vi "Open PDF.vi"(4 "error in (no error)":errorcluster, 7 "Path":path) -> (0 "error out":errorcluster, 2 "Cancelled":bool)   [LabVIEW 2015]
doc: "This VI opens a Acrobat Reader (.pdf) document in an external instance of Acrobat Reader.\nWire the path to the Acrobat Reader document to the Path input.\nIf this is left unwired this VI will prompt for the document."
uses:
  <vilib>/registry/registry.llb/Registry RtKey.ctl
  <vilib>/registry/registry.llb/Registry SAM.ctl
  <vilib>/registry/registry.llb/Read Registry Value Simple STR.vi
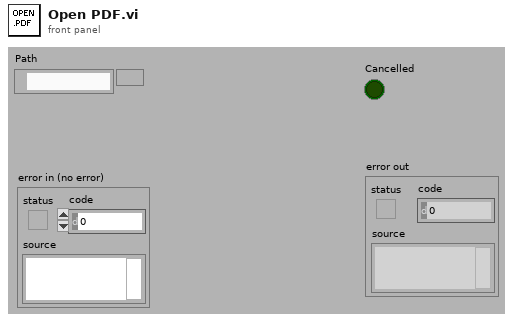
[diagram p1: front panel]
types:
  T1 = enum32{"existing file", "new file", "new or existing file", "existing dir", "new dir", "new or existing dir", "existing file (use LLBs)", "new file (use LLBs)", "new or existing file (use LLBs)", "new or existing file or directory (use LLBs)"}
  T2 = typedef "Registry SAM.ctl" = enum32{"KEY_QUERY_VALUE", "KEY_SET_VALUE", "KEY_CREATE_SUB_KEY", "KEY_ENUMERATE_SUB_KEYS", "KEY_NOTIFY", "KEY_CREATE_LINK", "KEY_READ", "KEY_WRITE", "KEY_ALL_ACCESS", "KEY_READ | KEY_WRITE"}
  T3 = typedef "Registry RtKey.ctl" = enum32{"HKEY_CLASSES_ROOT", "HKEY_CURRENT_USER", "HKEY_LOCAL_MACHINE", "HKEY_USERS", "HKEY_PERFORMANCE_DATA", "HKEY_CURRENT_CONFIG", "HKEY_DYN_DATA"}
  T4 = typedef "Registry refnum.ctl" = refnum<k1>
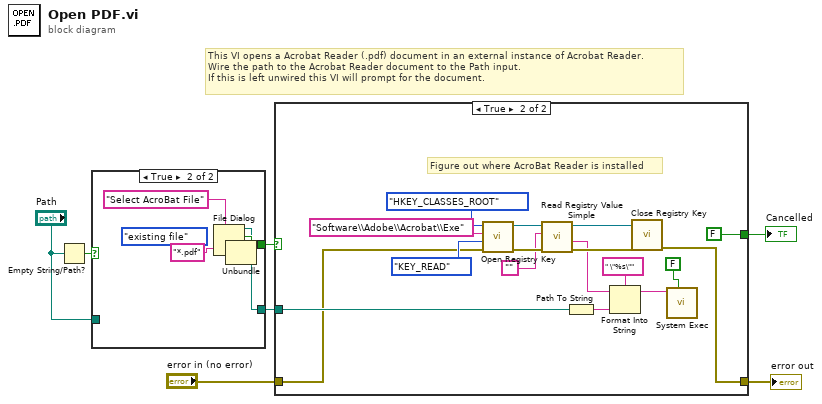
[diagram p0: block diagram]
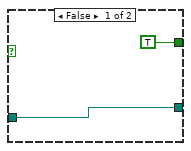
[diagram p2: hidden frame]
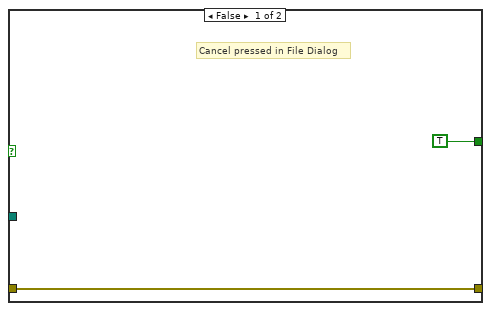
[diagram p3: hidden frame]
diagram:
  # "This VI opens a Acrobat Reader (.pdf) document in an external instance of Acrobat Reader.\nWire the path to the Acrobat Reader document to the Path input.\nIf this is left unwired this VI will prompt for the document."
  n1 = Empty String/Path?(string/path="Path") -> (empty?=w5:bool)
  n2 = case shown="True" w5 {
    tunnel: [TRUE ("exists") w12] -> w7
    tunnel: [w8 w11] -> w6
    tunnel: "Path" -> [w8 _]
    frame False {
    }
    frame True {
      (unwired) T1."existing file" ("select mode (2)")
      n3 = File Dialog(6:"*.pdf" ("pattern"), 7:"Select AcroBat File" ("prompt")) -> (0:w10:errorcluster, 2:w12:bool, 3:w11:path)  [unwired: 5 in, 1 out]
      n4 = Unbundle(w10) -> ()  [unwired: 3 out]
    }
  }
  n5 = case shown="True" w7 {
    tunnel: w6 -> [_ w20]
    tunnel: "error in (no error)" -> [w16 w19]
    tunnel: [w16 w18] -> w2
    tunnel: [TRUE FALSE] -> w1
    frame False {
      # "Cancel pressed in File Dialog"
    }
    frame True {
      # "Figure out where AcroBat Reader is installed"
      n6 = call <vilib>:"Open Registry Key.vi"("error in (no error)"=w19, "security access mask (KEY_READ | KEY_WRITE)"=Registry_SAM."KEY_READ", "subkey"="Software\\Adobe\\Acrobat\\Exe", "root key (HKEY_LOCAL_MACHINE)"=Registry_RtKey."HKEY_CLASSES_ROOT") -> ("error out"=w30:errorcluster, "refnum out"=w31:T4)  [unwired: 6 in]
      n7 = call-poly <vilib>:"Read Registry Value Simple.vi"("error in (no error)"=w30, "value"="", "refnum"=w31) -> ("error out"=w27:errorcluster, "String/Binary data"=w21:string, "refnum out"=w26:T4)  [unwired: 3 in, 1 out]
      n8 = Path To String(path=w20) -> (string=w24:string)
      n9 = Format Into String(format string=" \"%s\"", initial string=w21, w24) -> (resulting string=w22:string)  [unwired: 1 in, 1 out]
      n10 = call <vilib>:"Close Registry Key.vi"("error in (no error)"=w27, "refnum"=w26) -> ("error out"=w18:errorcluster)  [unwired: 5 in]
      n11 = call <vilib>:"System Exec.vi"("wait until completion? (T)"=FALSE, "command line"=w22) -> ()  [unwired: 6 in, 4 out]
    }
  }
  "error out" <- w2
  "Cancelled" <- w1
